vi "Track Rotation.vi"(8 "Angle Limiter":enum16{"90", "45", "15", "1"}(ring), 10 "Coord":cluster{dbl, dbl}, 11 "Point in":cluster{"x":dbl, "y":dbl, "th":dbl}) -> (3 "Point out":cluster{"x":dbl, "y":dbl, "th":dbl})   [LabVIEW 2019]
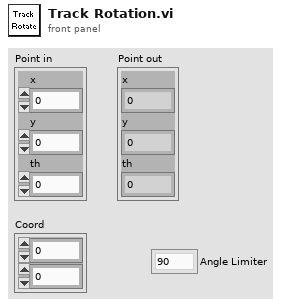
[diagram p1: front panel]
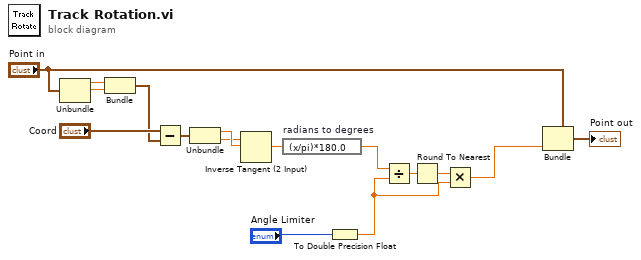
[diagram p0: block diagram]
diagram:
  n1 = Unbundle("Point in") -> ("x"=w13:dbl, "y"=w12:dbl)  [unwired: 1 out]
  n2 = Bundle("x"=w13, "y"=w12) -> (w11:cluster{"x":dbl, "y":dbl})  [unwired: 1 in]
  n3 = Subtract(x="Coord", y=w11) -> (x-y=w10:cluster{dbl, dbl})
  n4 = Unbundle(w10) -> (w9:dbl, w8:dbl)
  n5 = Inverse Tangent (2 Input)(1:w9, 2:w8) -> (0:w7:dbl)
  n6 = expression code="(x/pi)*180.0" "radians to degrees"(w7) -> (w4:dbl)
  n7 = To Double Precision Float(number="Angle Limiter") -> (double precision float=w1:dbl)
  n8 = Divide(x=w4, y=w1) -> (x/y=w6:dbl)
  n9 = Round To Nearest(number=w6) -> (nearest integer value=w5:dbl)
  n10 = Multiply(x=w5, y=w1) -> (x*y=w3:dbl)
  n11 = Bundle(cluster="Point in", "th"=w3) -> (→"Point out":cluster{"x":dbl, "y":dbl, "th":dbl})  [unwired: 2 in]
